vi "Scale.vi"(8 "error in (no error)":errorcluster, 10 "Scale":cluster{"X":dbl, "Y":dbl}={"X"=1.0, "Y"=1.0}, 11 "Static Image Transform in":refnum<class "Static Image Transform.lvclass">) -> (0 "error out":errorcluster, 3 "Static Image Transform out":refnum<class "Static Image Transform.lvclass">)   [LabVIEW 2020, in "Glyph Drawer.lvlib" / "Static Image Transform.lvclass"]
uses:
  Static Image Transform.lvclass
  Static Image Transform.lvclass/Static Image Transform.ctl
  <vilib>/Analysis/Matrix/Datatypes/RealMatrix.ctl
  <vilib>/Analysis/baseanly.llb/Real A x B.vi
  Glyph Drawer.lvlib
  <vilib>/Analysis/Matrix/NI_Matrix.lvlib
  <vilib>/Analysis/NI_AALBase.lvlib
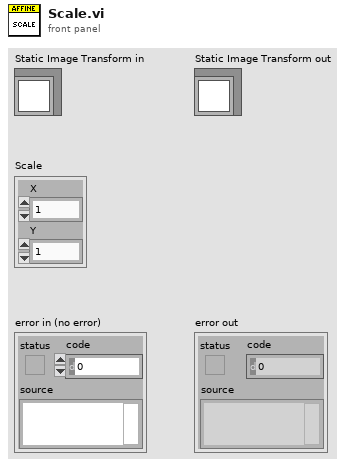
[diagram p1: front panel]
types:
  T1 = typedef "NI_Matrix.lvlib/RealMatrix.ctl" = dbl[][]
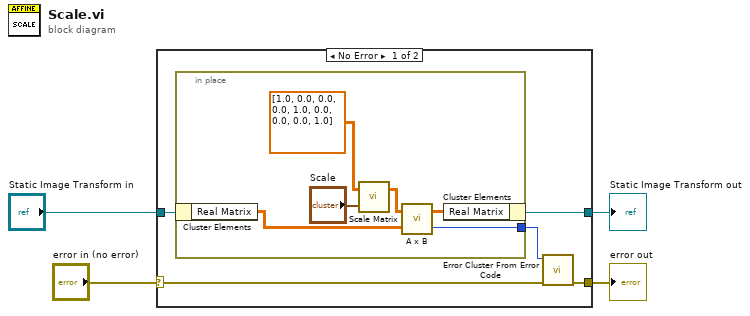
[diagram p0: block diagram]
diagram:
  n1 = case shown="No Error" "error in (no error)" {
    selector: "error in (no error)" -> [w8 w17]
    tunnel: [w6 w17] -> w3
    tunnel: [w7 w16] -> w1
    tunnel: "Static Image Transform in" -> [w9 w16]
    frame No Error {
      n2 = in-place {
        in-place-border: [w10] -> w5
        n3 = in-place-cluster #1(w9) -> ("Real Matrix"=w12:T1)
        n4 = call "Scale Matrix.vi"("Scale"="Scale", "Matrix Type (2x2)"=T1 [[1.0, 0.0, 0.0], [0.0, 1.0, 0.0], [0.0, 0.0, 1.0]]) -> ("Matrix Out"=w13:T1)  [unwired: 1 in]
        n5 = call-poly <vilib>:"A x B.vi"("B"=w12, "A"=w13) -> ("error"=w10:i32, "A x B"=w11:T1)
        n6 = in-place-cluster #1("Real Matrix"=w11) -> (w7:refnum<class "Static Image Transform.lvclass">)
      }
      n7 = call <vilib>:"Error Cluster From Error Code.vi"("error in (no error)"=w8, "error code (0)"=w5) -> ("error out"=w6:errorcluster)  [unwired: 7 in]
    }
    frame Error {
    }
  }
  "error out" <- w3
  "Static Image Transform out" <- w1
